vi "Pulse Stretch & Delay Demonstrator.vi"() -> ()   [LabVIEW 2011]
panel:
  out "Table":string[][](table)
  in  "Width (sec)":dbl=1.0
  out "Out":bool
  in  "Delay (sec)":dbl=1.0
  in  "In":bool
  # "D,W\n0,0 makes one-iteration pulse\npos, 0 makes no pulse"
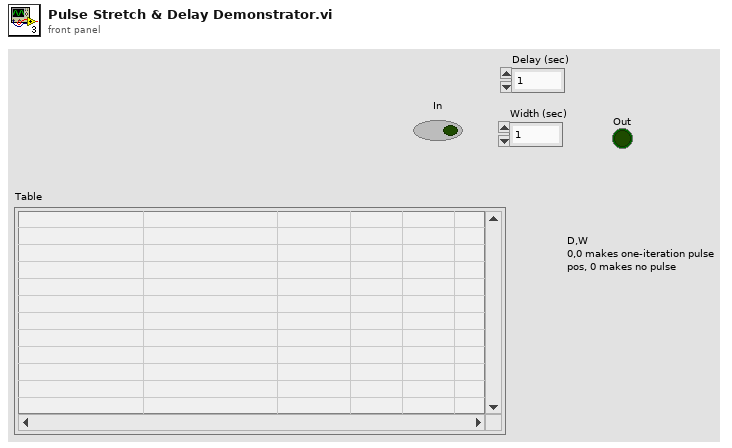
[diagram p1: front panel]
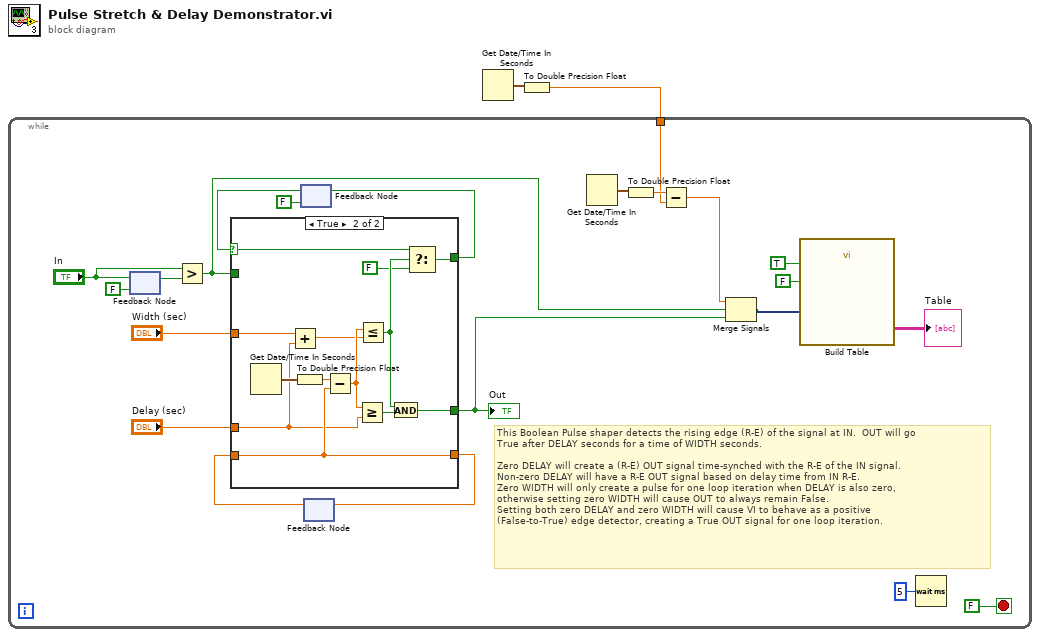
[diagram p0: block diagram]
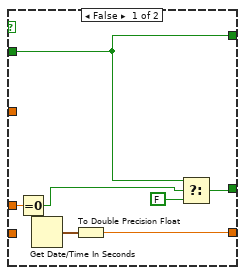
[diagram p2: hidden frame]
diagram:
  n1 = Get Date/Time In Seconds() -> (seconds since 1Jan1904=w2:timestamp)
  n2 = To Double Precision Float(number=w2) -> (double precision float=w1:dbl)
  n3 = while {
    tunnel: w1 -> [w3]
    stop <- FALSE stop-if-true
    # "This Boolean Pulse shaper detects the rising edge (R-E) of the signal at IN.  OUT will go\nTrue after DELAY seconds for a time of WIDTH seconds. \n\nZero DELAY will create a (R-E) OUT signal time-synched with the R-E of the IN signal.\nNon-zero DELAY will have a R-E OUT signal based on delay time from IN R-E.\nZero WIDTH will only create a pulse for one loop iteration when DELAY is also zero,\notherwise setting zero WIDTH will cause OUT to always remain False.\nSetting both zero DELAY and zero WIDTH will cause VI to behave as a positive\n(False-to-True) edge detector, creating a True OUT signal for one loop iteration."
    n4 = feedback #1(FALSE ("input")) -> (w23:bool)
    n5 = feedback-in #1("In") -> ()
    n6 = Greater?(x="In", y=w23) -> (0:w6:bool)
    n7 = feedback #2(FALSE) -> (w18:bool)
    n8 = feedback #3() -> (w20:dbl)  [unwired: 1 in]
    n9 = case shown="True" w18 {
      selector: w18 -> [_ w35]
      tunnel: [w30 w39] -> w21
      tunnel: w20 -> [_ w39]
      tunnel: [w28 w43] -> w19
      tunnel: w6 -> [w28 _]
      tunnel: [w27 w40] -> w5
      tunnel: "Delay (sec)" -> [w29 w33]
      tunnel: "Width (sec)" -> [_ w32]
      frame False {
        n10 = Equal To 0?(x=w29) -> (x = 0?=w25:bool)
        n11 = Get Date/Time In Seconds() -> (seconds since 1Jan1904=w31:timestamp)
        n12 = To Double Precision Float(number=w31) -> (double precision float=w30:dbl)
        n13 = Select(t=w28, s=w25, f=FALSE) -> (s? t:f=w27:bool)
      }
      frame True {
        n14 = Get Date/Time In Seconds() -> (seconds since 1Jan1904=w44:timestamp)
        n15 = Add(x=w32, y=w33) -> (x+y=w37:dbl)
        n16 = To Double Precision Float(number=w44) -> (double precision float=w41:dbl)
        n17 = Subtract(x=w41, y=w39) -> (x-y=w38:dbl)
        n18 = Greater Or Equal?(x=w38, y=w33) -> (x >= y?=w42:bool)
        n19 = Less Or Equal?(x=w38, y=w37) -> (x <= y?=w36:bool)
        n20 = And(x=w36, y=w42) -> (x .and. y?=w40:bool)
        n21 = Select(t=w35, s=w36, f=FALSE) -> (s? t:f=w43:bool)
      }
    }
    "Out" <- w5
    n22 = feedback-in #2(w19) -> ()
    n23 = feedback-in #3(w21) -> ()
    n24 = Get Date/Time In Seconds() -> (seconds since 1Jan1904=w11:timestamp)
    n25 = To Double Precision Float(number=w11) -> (double precision float=w10:dbl)
    n26 = Subtract(x=w10, y=w3) -> (x-y=w9:dbl)
    n27 = Merge Signals(w9, w6, w5) -> (w12:dynamicdata)
    n28 = call "Build Table"("Include time data"=FALSE, "Enable"=TRUE, "Signals"=w12) -> ("Table"=→"Table":string[][])  [unwired: 2 in, 6 out]
    n29 = Wait (ms)(milliseconds to wait=u32 5) -> ()  [unwired: 1 out]
  }
